vi "Cast Data Class.vi"(8 "error in":errorcluster, 10 "Type":string, 11 "Alicat Device in":refnum<class "Alicat Device.lvclass">) -> (0 "error out":errorcluster, 2 "Alicat Data Out":refnum<class "Alicat Data.lvclass">, 3 "Alicat Device out":refnum<class "Alicat Device.lvclass">)   [LabVIEW 2015, in "Alicat Lib.lvlib" / "Alicat Device.lvclass"]
doc: "Load the data class dynamically. If the class can not be found, load the default class (Alicat Data) so everything does not break."
uses:
  Alicat Device.lvclass
  Data/Alicat Data.lvclass
  <vilib>/MSR Consulting, LLC/Configurable Device/Configurable Device.lvclass/Configurable Device.ctl
  Alicat Device.lvclass/Alicat Device.ctl
  Data/Alicat Data.lvclass/Alicat Data.ctl
  <vilib>/MSR Consulting, LLC/Configurable Device/Accessors/Write controller_.vi
  Accessors/Read Alicat Data.vi
  Data/Write Alicat ype.vi
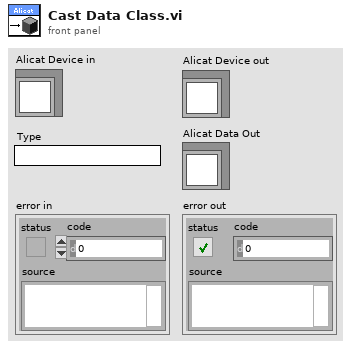
[diagram p1: front panel]
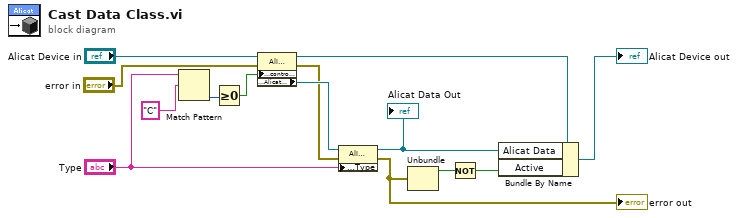
[diagram p0: block diagram]
diagram:
  n1 = Match Pattern(string="Type", regular expression="C") -> (offset past match=w13:i32)  [unwired: 1 in, 3 out]
  n2 = Greater Or Equal To 0?(x=w13) -> (x >= 0?=w6:bool)
  n3 = property class="Alicat Device"(reference="Alicat Device in", error in="error in", "Accessors:controller_"=w6) -> (reference out=w7:refnum<class "Alicat Device.lvclass">, error out=w1:errorcluster, "Accessors:Alicat Data"=w5:refnum<class "Alicat Data.lvclass">)
  n4 = property class="Alicat Data"(reference=w5, error in=w1, "Accessors:Type"="Type") -> (reference out=w11:refnum<class "Alicat Data.lvclass">, error out=w4:errorcluster)
  "error out" <- w4
  "Alicat Data Out" <- w11
  n5 = Unbundle(w4) -> ("status"=w10:bool)  [unwired: 2 out]
  n6 = Not(x=w10) -> (.not. x?=w3:bool)
  n7 = Bundle By Name(cluster=w7, "Alicat Data"=w11, "Active"=w3) -> (→"Alicat Device out":refnum<class "Alicat Device.lvclass">)
